vi "TestCOM.vi"() -> ()   [LabVIEW 2011]
panel:
  out "Image":T1(plugin-control)
  out "Center of mass":cluster{"comX":sgl, "comY":sgl}
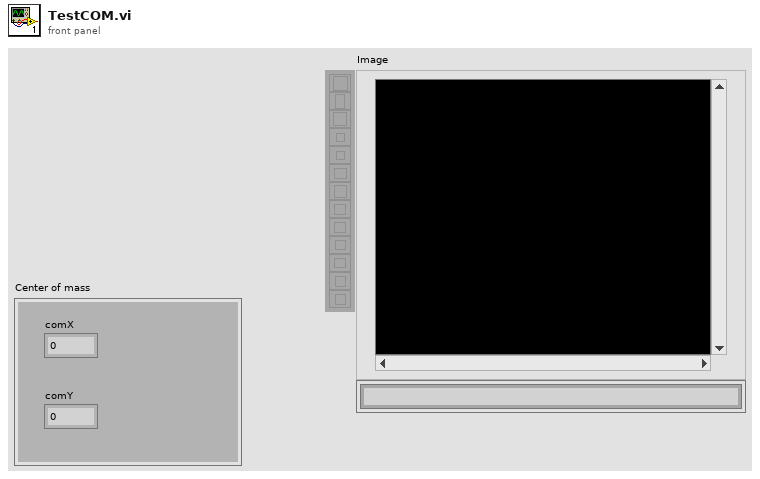
[diagram p1: front panel]
types:
  T1 = typedef "IMAQ Image.ctl" = refnum<image>
  T2 = typedef "Image Type" = u32
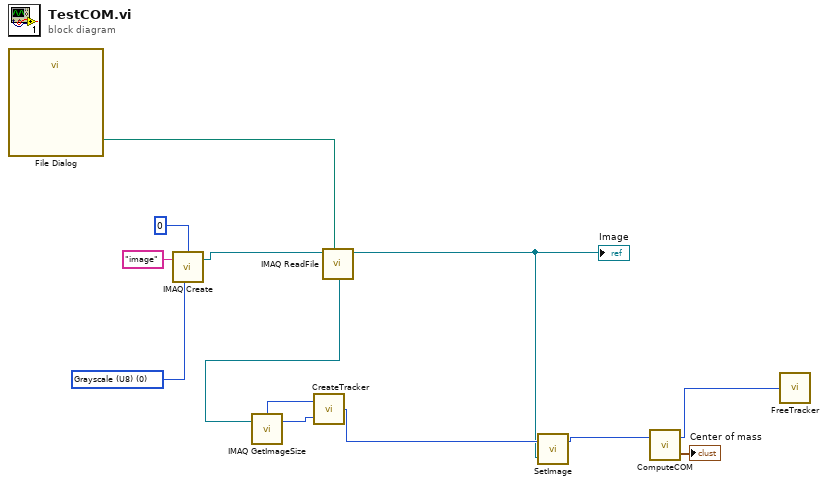
[diagram p0: block diagram]
diagram:
  w11 = T2 0 items=["Grayscale (U8)", "Grayscale (I16)", "Grayscale (SGL)", "Complex (CSG)", "RGB (U32)", "HSL (U32)", "RGB (U64)", "Grayscale (U16)"] ("Image Type")
  n1 = call "File Dialog"() -> ("selected path"=w4:path)  [unwired: 12 in, 3 out]
  n2 = call "IMAQ Create"("Border Size"=0, "Image Name"="image", "Image Type"=w11) -> ("New Image"=w9:T1)  [unwired: 2 in, 1 out]
  n3 = call "IMAQ ReadFile"("File Path"=w4, "Image"=w9) -> ("Image Out"=w3:T1)  [unwired: 5 in, 4 out]
  "Image" <- w3
  n4 = call "IMAQ GetImageSize"("Image"=w3) -> ("Y Resolution"=w1:i32, "X Resolution"=w2:i32)  [unwired: 3 in, 1 out]
  n5 = call "CreateTracker.vi"("height"=w1, "width"=w2) -> ("return type"=w8:u64)
  n6 = call "SetImage.vi"("image"=w3, "tracker"=w8) -> ("tracker"=w7:u64)  [unwired: 1 in]
  n7 = call "ComputeCOM.vi"("tracker"=w7) -> ("Center of mass"=→"Center of mass":cluster{"comX":sgl, "comY":sgl}, "tracker"=w5:u64)  [unwired: 1 in]
  n8 = call "FreeTracker.vi"("trackerInstance"=w5) -> ()
